vi "ReadXYandSensitivitySR5110.vi"(11 "7265 GPIB":string="7") -> (0 "Sen":dbl format="%#_13g", 2 "Yout":dbl format="%#_13g", 3 "Xout":dbl format="%#_13g")   [LabVIEW 2013]
panel:
  out "Xout 2":dbl format="%#_13g"
  out "Yout 2":dbl format="%#_13g"
  out "error out":errorcluster
  in  "error in (no error)":errorcluster
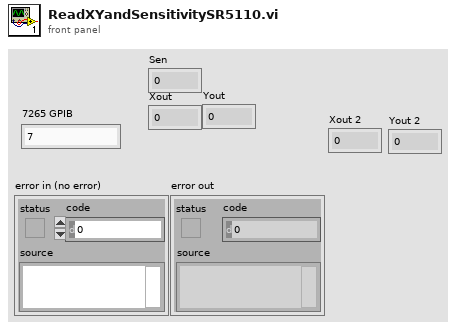
[diagram p1: front panel]
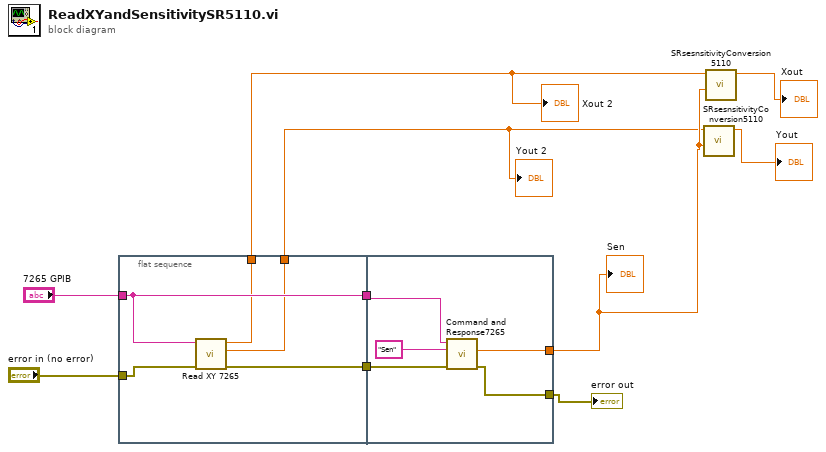
[diagram p0: block diagram]
diagram:
  n1 = flat-sequence {
    tunnel: "7265 GPIB" -> [w13]
    tunnel: "error in (no error)" -> [w15]
    tunnel: [w14] -> w7
    tunnel: [w13] -> w6
    tunnel: [w12] -> w2
    tunnel: [w11] -> w1
    tunnel: [w19] -> w10
    tunnel: w7 -> [w18]
    tunnel: w6 -> [w17]
    tunnel: [w16] -> w5
    frame #0 {
      n2 = call "Read XY 7265.vi"("error in (no error)"=w15, "7265 GPIB"=w13) -> ("error out"=w14:errorcluster, "Y channel"=w12:dbl, "X channel"=w11:dbl)  [unwired: 7 in]
    }
    frame #1 {
      n3 = call "Command and Response7265.vi"("error in (no error)"=w18, "Command"="Sen", "7265 GPIB"=w17) -> ("error out"=w19:errorcluster, "Response Code Only"=w16:dbl)  [unwired: 6 in, 1 out]
    }
  }
  n4 = call "SRsesnsitivityConversion5110.vi"("Sen"=w5, "Input"=w2) -> ("Output"=→"Yout":dbl)  [unwired: 9 in]
  n5 = call "SRsesnsitivityConversion5110.vi"("Sen"=w5, "Input"=w1) -> ("Output"=→"Xout":dbl)  [unwired: 9 in]
  "error out" <- w10
  "Sen" <- w5
  "Yout 2" <- w2
  "Xout 2" <- w1
